vi "AE - Bluetooth.vi"(7 "Enum":T1, 8 "error in (no error)":errorcluster, 11 "Variant In":variant) -> (0 "error out":errorcluster, 3 "Variant Out":variant, 4 "get_Item":refnum<k24>)   [LabVIEW 2010]
uses:
  AE - Bluetooth Enum.ctl
  C:/Users/×ñÞóôïò/Desktop/Systems real time/koupe proj/experiments 2/Resources/WiimoteLib.dll
  experiments 2/Resources/WiimoteLib.dll
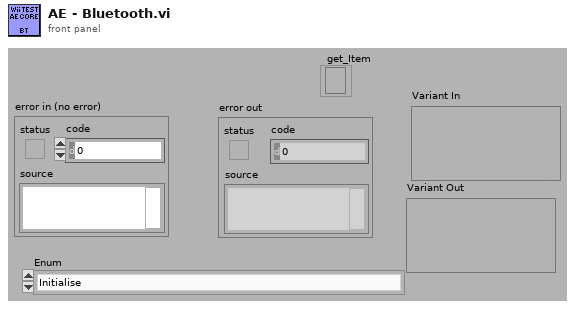
[diagram p1: front panel]
types:
  T1 = typedef "AE - Bluetooth Enum.ctl" = enum16{"Initialise", "Pair All Wiimotes", "Connect All Wiimotes", "Set Rumble", "Set LED", "Get Button + Acc Data", "Get IR Data", "Get Battery", "Get Wiimote Reference", "Reorder Wiimotes", "devReport"}
  T2 = typedef "wiimotestate.ctl" = cluster{"X":sgl, "Y":sgl, "Z":sgl, "A":bool, "B":bool, "Down":bool, "Home":bool, "Left":bool, "Minus":bool, "One":bool, "Plus":bool, "Right":bool, "Two":bool, "Up":bool, "error out":errorcluster}
  T3 = typedef "wiimoteState(IR).ctl" = cluster{"Mode":u8, "IR State":bool[], "X Values":sgl[], "Y Values":sgl[], "Raw X Values":i32[], "Raw Y Values":i32[], "Sizes":i32[], "X Midpoint":sgl, "Y Midpoint":sgl}
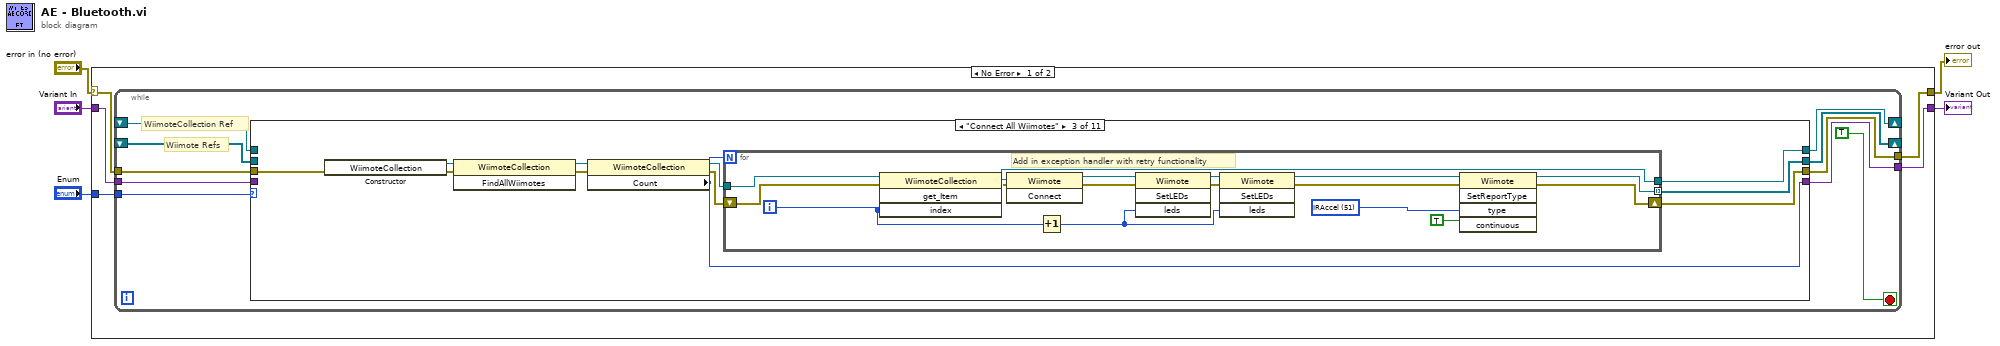
[diagram p0: block diagram]
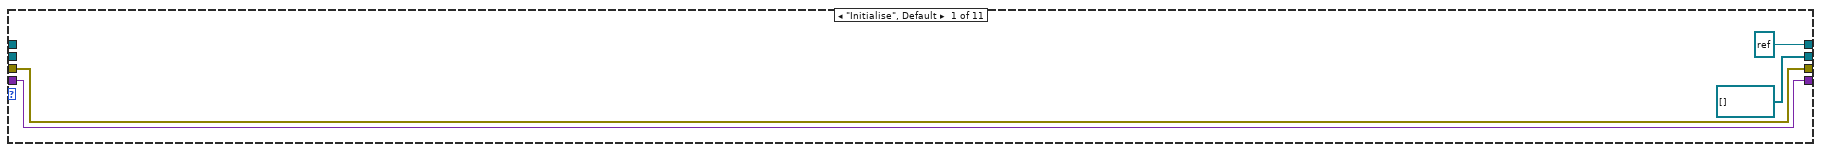
[diagram p2: hidden frame]
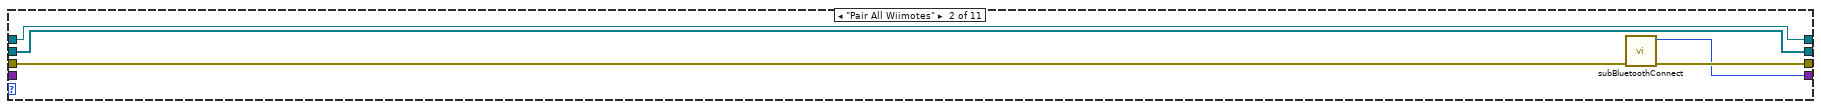
[diagram p3: hidden frame]
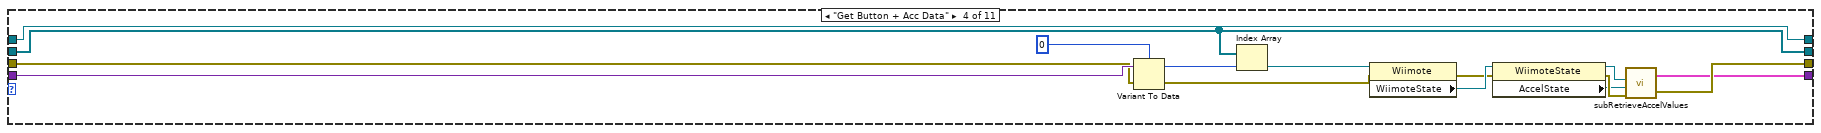
[diagram p4: hidden frame]
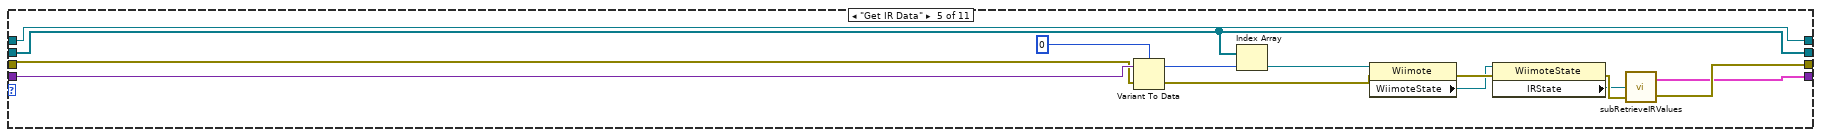
[diagram p5: hidden frame]
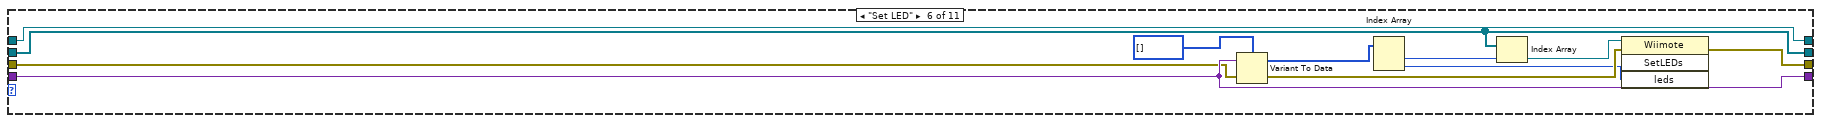
[diagram p6: hidden frame]
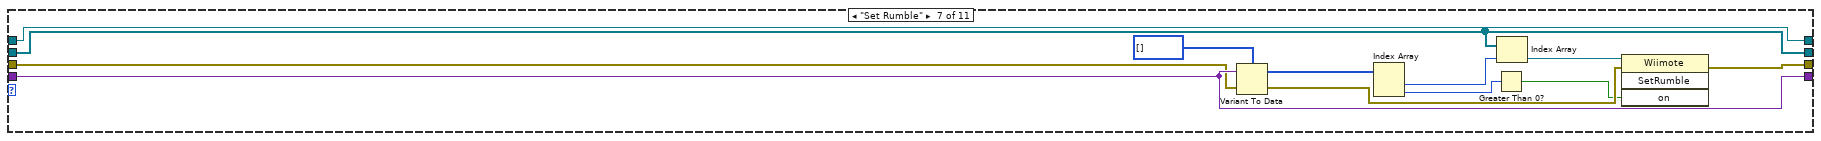
[diagram p7: hidden frame]
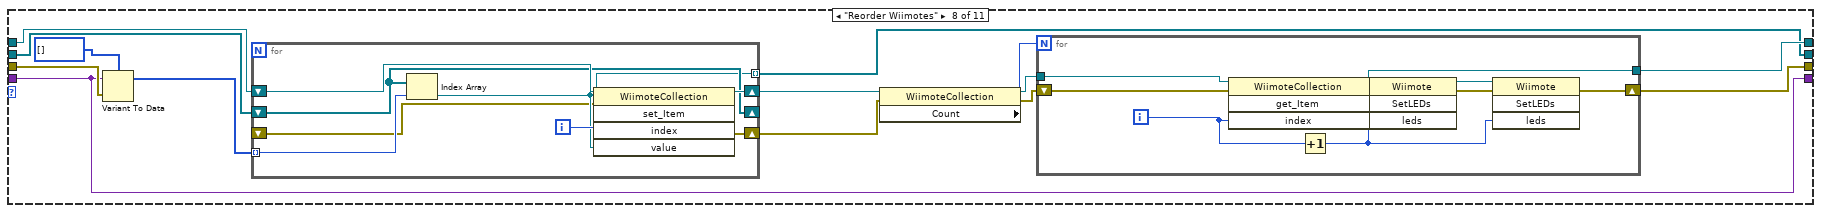
[diagram p8: hidden frame]
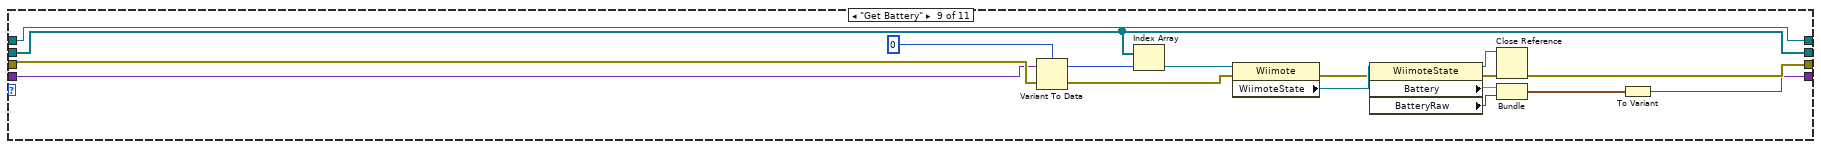
[diagram p9: hidden frame]
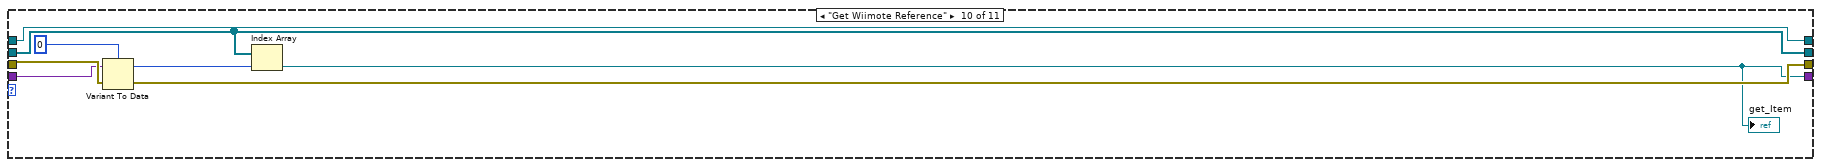
[diagram p10: hidden frame]
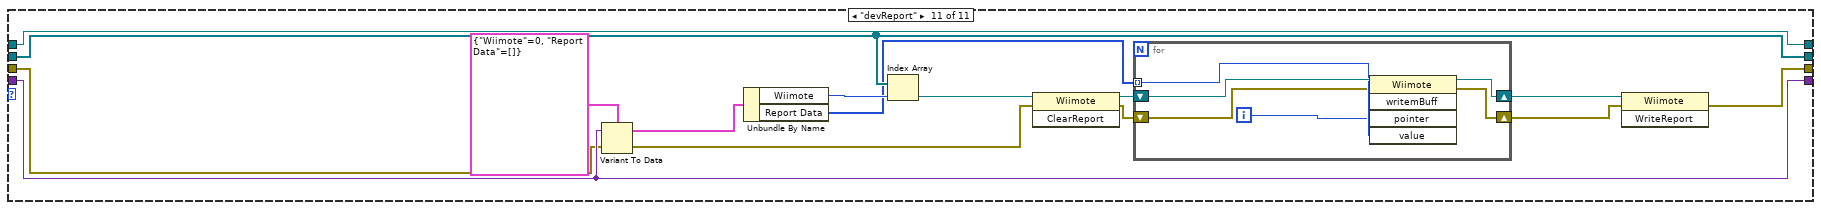
[diagram p11: hidden frame]
diagram:
  n1 = case shown="No Error" "error in (no error)" {
    selector: "error in (no error)" -> [w10 w189]
    tunnel: [w9 w189] -> w4
    tunnel: "Enum" -> [w8 _]
    tunnel: "Variant In" -> [w7 w188]
    tunnel: [w6 w188] -> w1
    frame No Error {
      n2 = while {
        tunnel: w10 -> [w19]
        tunnel: [w18] -> w9
        tunnel: w8 -> [w11]
        tunnel: w7 -> [w17]
        tunnel: [w16] -> w6
        shift-right: [w15] -> _
        shift-left: _ -> [w14]
        shift-right: [w13] -> _
        shift-left: _ -> [w12]
        stop <- TRUE stop-if-true
        # "Wiimote Refs"
        # "WiimoteCollection Ref"
        n3 = case shown="\"Connect All Wiimotes\"" w11 {
          tunnel: w19 -> [w24 w27 w34 w69 w78 w94 w101 w122 w155 w162 w178]
          tunnel: [w24 w26 w33 w66 w77 w88 w100 w120 w147 w161 w171] -> w18
          tunnel: w17 -> [w23 _ _ w70 w80 w96 w105 w121 w143 w160 w179]
          tunnel: [w23 w25 w32 w65 w73 w96 w105 w121 w142 w159 w179] -> w16
          tunnel: [refnum<k24> refnum ("new reference") w29 w31 w72 w86 w97 w109 w119 w158 w166 w181] -> w15
          tunnel: w14 -> [_ w29 _ w72 w86 w97 w109 w113 w158 w166 w181]
          tunnel: [refnum<k24>[] [] w28 w30 w58 w76 w92 w104 w110 w154 w164 w180] -> w13
          tunnel: w12 -> [_ w28 _ w58 w76 w92 w104 w115 w154 w164 w180]
          frame "Initialise", Default {
          }
          frame "Pair All Wiimotes" {
            n4 = call "subBluetoothConnect.vi"("error in (no error)"=w27) -> ("error out"=w26:errorcluster, "Number of Wiimotes Connected"=w25:i32)  [unwired: 8 in, 1 out]
          }
          frame "Connect All Wiimotes" {
            n5 = constructor class="WiimoteCollection"(error in=w34) -> (reference out=w40:refnum<k24>, error out=w39:errorcluster)  [unwired: 2 in, 1 out]
            n6 = invoke class="WiimoteCollection" method="FindAllWiimotes"(reference=w40, error in=w39) -> (reference out=w38:refnum<k24>, error out=w37:errorcluster)  [unwired: 1 in, 1 out]
            n7 = property class="WiimoteCollection"(reference=w38, error in=w37) -> (reference out=w36:refnum<k24>, error out=w35:errorcluster, "Count"=w32:i32)
            n8 = for {
              N: w32 -> [_]
              tunnel: w36 -> [w55]
              shift-right: [w47] -> w33
              shift-left: w35 -> [w57]
              tunnel: [w56] -> w31
              tunnel: [w48] -> w30 mode=indexing
              i -> [w52]
              w54 = u8 51 items=["Status"=32, "ReadData"=33, "Buttons"=48, "ButtonsAccel"=49, "IRAccel"=51, "ButtonsExtension"=52, "ExtensionAccel"=53, "IRExtensionAccel"=55] ("type")
              # "Add in exception handler with retry functionality"
              n9 = invoke class="WiimoteCollection" method="get_Item"(reference=w55, error in=w57, "index"=w52) -> (reference out=w56:refnum<k24>, error out=w50:errorcluster, "get_Item"=w51:refnum<k24>)  [unwired: 1 in, 1 out]
              n10 = invoke class="Wiimote" method="Connect"(reference=w51, error in=w50) -> (reference out=w49:refnum<k24>, error out=w46:errorcluster)  [unwired: 1 in, 1 out]
              n11 = Increment(x=w52) -> (x+1=w41:i32)
              n12 = invoke class="Wiimote" method="SetLEDs"(reference=w49, error in=w46, "leds"=w41) -> (reference out=w45:refnum<k24>, error out=w44:errorcluster)  [unwired: 1 in, 2 out]
              n13 = invoke class="Wiimote" method="SetLEDs"(reference=w45, error in=w44, "leds"=w41) -> (reference out=w42:refnum<k24>, error out=w43:errorcluster)  [unwired: 1 in, 2 out]
              n14 = invoke class="Wiimote" method="SetReportType"(reference=w42, error in=w43, "type"=w54, "continuous"=TRUE) -> (reference out=w48:refnum<k24>, error out=w47:errorcluster)  [unwired: 1 in, 3 out]
            }
          }
          frame "Get Button + Acc Data" {
            n15 = Variant To Data(error in=w69, Variant=w70, type=0) -> (error out=w67:errorcluster, data=w68:i32)
            n16 = Index Array(array=w58, index=w68) -> (element=w59:refnum<k24>)
            n17 = property class="Wiimote"(reference=w59, error in=w67) -> (error out=w60:errorcluster, "WiimoteState"=w61:refnum<k24>)  [unwired: 1 out]
            n18 = property class="WiimoteState"(reference=w61, error in=w60) -> (reference out=w62:refnum<k24>, error out=w64:errorcluster, "AccelState"=w63:refnum<k24>)
            n19 = call "subRetrieveAccelValues.vi"("error in"=w64, "AccelState"=w63, "WiimoteState"=w62) -> ("error out"=w66:errorcluster, "Wiimote State"=w65:T2)  [unwired: 1 in]
          }
          frame "Get IR Data" {
            n20 = Variant To Data(error in=w78, Variant=w80, type=0) -> (error out=w79:errorcluster, data=w75:i32)
            n21 = Index Array(array=w76, index=w75) -> (element=w74:refnum<k24>)
            n22 = property class="Wiimote"(reference=w74, error in=w79) -> (error out=w85:errorcluster, "WiimoteState"=w84:refnum<k24>)  [unwired: 1 out]
            n23 = property class="WiimoteState"(reference=w84, error in=w85) -> (error out=w83:errorcluster, "IRState"=w82:refnum<k24>)  [unwired: 1 out]
            n24 = call "subRetrieveIRValues.vi"("error in"=w83, "IRState"=w82) -> ("error out"=w77:errorcluster, "IRState"=w73:T3)  [unwired: 1 in]
          }
          frame "Set LED" {
            n25 = Variant To Data(error in=w94, Variant=w96, type=u8[] []) -> (error out=w89:errorcluster, data=w93:u8[])
            n26 = Index Array(array=w93) -> (element #1=w91:u8, element #2=w87:u8)  [unwired: 2 in]
            n27 = Index Array(array=w92, index=w91) -> (element=w90:refnum<k24>)
            n28 = invoke class="Wiimote" method="SetLEDs"(reference=w90, error in=w89, "leds"=w87) -> (error out=w88:errorcluster)  [unwired: 1 in, 3 out]
          }
          frame "Set Rumble" {
            n29 = Variant To Data(error in=w101, Variant=w105, type=u8[] []) -> (error out=w102:errorcluster, data=w107:u8[])
            n30 = Index Array(array=w107) -> (element #1=w106:u8, element #2=w99:u8)  [unwired: 2 in]
            n31 = Greater Than 0?(x=w99) -> (x > 0?=w98:bool)
            n32 = Index Array(array=w104, index=w106) -> (element=w103:refnum<k24>)
            n33 = invoke class="Wiimote" method="SetRumble"(reference=w103, error in=w102, "on"=w98) -> (error out=w100:errorcluster)  [unwired: 1 in, 3 out]
          }
          frame "Reorder Wiimotes" {
            n34 = Variant To Data(error in=w122, Variant=w121, type=i32[] []) -> (data=w114:i32[])  [unwired: 1 out]
            n35 = for {
              shift-right: [w127] -> _
              shift-left: w115 -> [w127]
              tunnel: w114 -> [w130] mode=indexing
              shift-right: [w128] -> w112
              shift-left: w113 -> [w129]
              tunnel: [w126] -> w110 mode=indexing
              shift-right: [w125] -> w111
              shift-left: _ -> [w124]
              i -> [w131]
              n36 = Index Array(array=w127, index=w130) -> (element=w126:refnum<k24>)
              n37 = invoke class="WiimoteCollection" method="set_Item"(reference=w129, error in=w124, "index"=w131, "value"=w126) -> (reference out=w128:refnum<k24>, error out=w125:errorcluster)  [unwired: 1 in, 3 out]
            }
            n38 = property class="WiimoteCollection"(reference=w112, error in=w111) -> (reference out=w118:refnum<k24>, error out=w116:errorcluster, "Count"=w117:i32)
            n39 = for {
              N: w117 -> [_]
              shift-right: [w136] -> w120
              shift-left: w116 -> [w134]
              tunnel: [w141] -> w119
              tunnel: w118 -> [w132]
              i -> [w140]
              n40 = invoke class="WiimoteCollection" method="get_Item"(reference=w132, error in=w134, "index"=w140) -> (reference out=w141:refnum<k24>, error out=w135:errorcluster, "get_Item"=w133:refnum<k24>)  [unwired: 1 in, 1 out]
              n41 = Increment(x=w140) -> (x+1=w137:i32)
              n42 = invoke class="Wiimote" method="SetLEDs"(reference=w133, error in=w135, "leds"=w137) -> (reference out=w139:refnum<k24>, error out=w138:errorcluster)  [unwired: 1 in, 2 out]
              n43 = invoke class="Wiimote" method="SetLEDs"(reference=w139, error in=w138, "leds"=w137) -> (error out=w136:errorcluster)  [unwired: 1 in, 3 out]
            }
          }
          frame "Get Battery" {
            n44 = Variant To Data(error in=w155, Variant=w143, type=u8 0) -> (error out=w152:errorcluster, data=w156:u8)
            n45 = Index Array(array=w154, index=w156) -> (element=w153:refnum<k24>)
            n46 = property class="Wiimote"(reference=w153, error in=w152) -> (error out=w148:errorcluster, "WiimoteState"=w151:refnum<k24>)  [unwired: 1 out]
            n47 = property class="WiimoteState"(reference=w151, error in=w148) -> (reference out=w150:refnum<k24>, error out=w149:errorcluster, "Battery"=w146:sgl, "BatteryRaw"=w145:u8)
            n48 = Close Reference(reference=w150, error in (no error)=w149) -> (error out=w147:errorcluster)
            n49 = Bundle("Battery"=w146, "BatteryRaw"=w145) -> (w144:cluster{"Battery":sgl, "BatteryRaw":u8})  [unwired: 1 in]
            n50 = To Variant(anything=w144) -> (Variant=w142:variant)
          }
          frame "Get Wiimote Reference" {
            n51 = Variant To Data(error in=w162, Variant=w160, type=u8 0) -> (error out=w161:errorcluster, data=w163:u8)
            n52 = Index Array(array=w164, index=w163) -> (element=w159:refnum<k24>)
            "get_Item" <- w159
          }
          frame "devReport" {
            n53 = Variant To Data(error in=w178, Variant=w179, type=cluster{"Wiimote":u8, "Report Data":u8[]} {"Wiimote"=0, "Report Data"=[]}) -> (error out=w172:errorcluster, data=w169:cluster{"Wiimote":u8, "Report Data":u8[]})
            n54 = Unbundle By Name(w169) -> ("Wiimote"=w168:u8, "Report Data"=w167:u8[])
            n55 = Index Array(array=w180, index=w168) -> (element=w177:refnum<k24>)
            n56 = invoke class="Wiimote" method="ClearReport"(reference=w177, error in=w172) -> (reference out=w176:refnum<k24>, error out=w174:errorcluster)  [unwired: 1 in, 1 out]
            n57 = for {
              shift-right: [w186] -> w175
              shift-left: w176 -> [w187]
              tunnel: w167 -> [w185] mode=indexing
              shift-right: [w182] -> w173
              shift-left: w174 -> [w183]
              i -> [w184]
              n58 = invoke class="Wiimote" method="writemBuff"(reference=w187, error in=w183, "pointer"=w184, "value"=w185) -> (reference out=w186:refnum<k24>, error out=w182:errorcluster)  [unwired: 1 in, 3 out]
            }
            n59 = invoke class="Wiimote" method="WriteReport"(reference=w175, error in=w173) -> (error out=w171:errorcluster)  [unwired: 1 in, 2 out]
          }
        }
      }
    }
    frame Error {
    }
  }
  "error out" <- w4
  "Variant Out" <- w1
